vi "RPM probe test.vi"() -> ()   [LabVIEW 2016]
doc: "This example demonstrates how to write time-domain and frequency-domain data to a TDMS file using the Write to Measurement File Express VI."
uses:
  <vilib>/express/express analysis/Spectral/Block/exnSpectralBlock spectral measurements power poly.vi
  <vilib>/express/express analysis/Spectral/Block/exnSpectralBlock spectral measurements power DDT.vi
  <vilib>/express/express analysis/Spectral/XNode/ExpressSpectralMeasurementsBlockNode.xnode
panel:
  out "Boolean":bool
  in  "Dial":dbl(knob) scale=0.0..6500.0
  out "Measured Data":dynamicdata(graph)
  out "Power Spectrum":dynamicdata(graph)
  out "Scan number":i32
  in  "Stop":bool
  out "Value 2":i32 format="%_5f"
  # "Overview: Demonstrates how to write time-domain and frequency-domain data to a TDMS file using the Write to Measurement File Express VI.\nInstructions:\n1. Run the VI.\n2. Click Stop to stop the VI. The TDMS file will be displayed in the TDMS File Viewer.\n3. Delete the .tdms file (located at [LabVIEW Data]\\Example Time And Frequency Domain.tdms) when you are done."
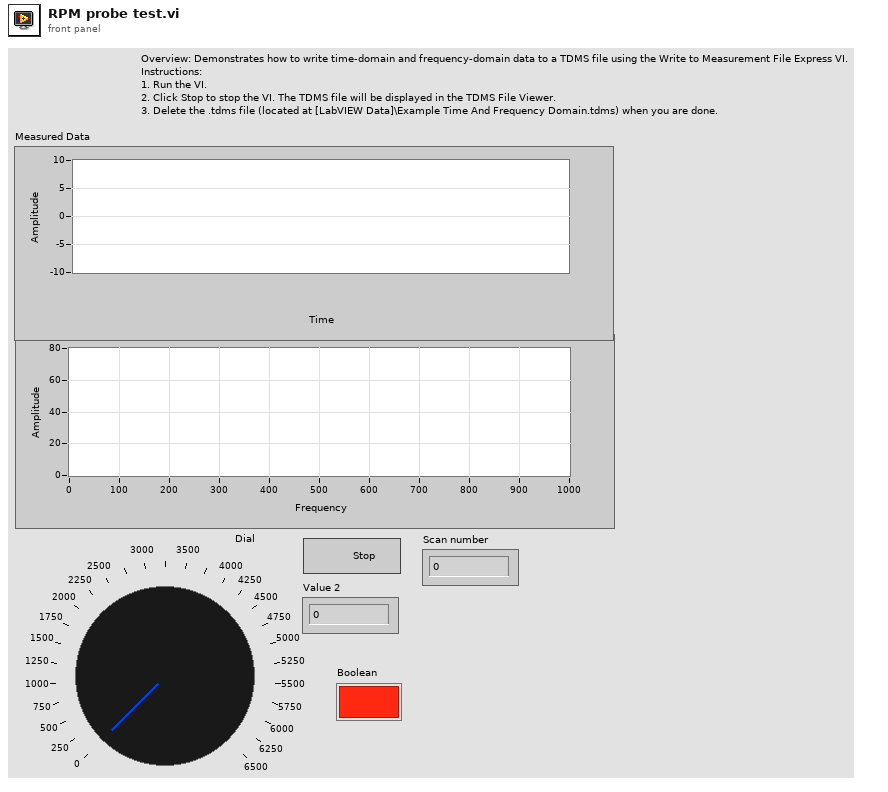
[diagram p1: front panel]
types:
  T1 = cluster{"averaging mode":u16, "weighting mode":u16, "number of averages":u32}
  T2 = cluster{"dB On (F)":bool, "unwrap phase (F)":bool, "convert to degree (F)":bool}
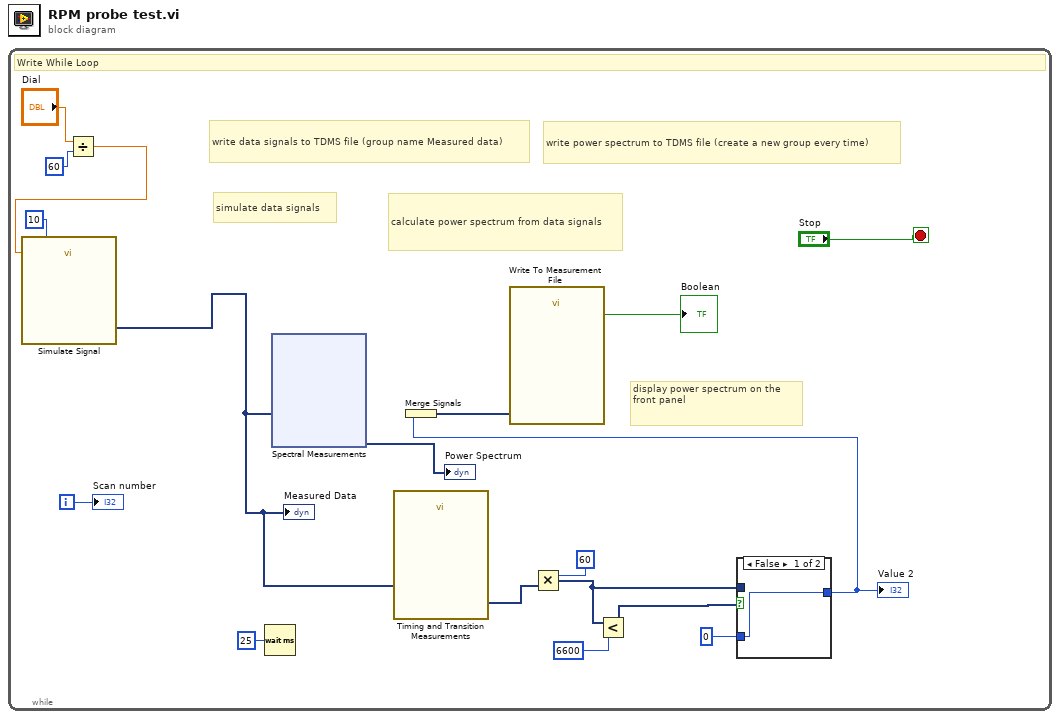
[diagram p0: block diagram]
diagram:
  n1 = while {
    i -> [w18]
    stop <- "Stop" stop-if-true
    # "simulate data signals"
    # "display power spectrum on the front panel"
    # "write power spectrum to TDMS file (create a new group every time)"
    # "calculate power spectrum from data signals"
    # "write data signals to TDMS file (group name Measured data)"
    # "Write While Loop"
    n2 = Divide(x="Dial", y=u32 60 ("milliseconds to wait")) -> (x/y=w6:dbl)
    n3 = call "Simulate Signal"("Frequency"=w6, "Amplitude"=u32 10 ("milliseconds to wait")) -> ("Square"=w11:dynamicdata)  [unwired: 5 in, 8 out]
    "Measured Data" <- w11
    n4 = Wait (ms)(milliseconds to wait=u32 25) -> ()  [unwired: 1 out]
    n5 = xnode "Spectral Measurements"("Signals"=w11) -> ("Power Spectrum"=→"Power Spectrum":dynamicdata)  [unwired: 1 in, 1 out]
    n6 = call "Timing and Transition Measurements"("Signals"=w11) -> ("Frequency"=w15:dynamicdata)  [unwired: 9 in, 1 out]
    n7 = Multiply(x=u32 60 ("milliseconds to wait"), y=w15) -> (x*y=w2:dynamicdata)
    n8 = Less?(x=w2, y=u32 6600 ("milliseconds to wait")) -> (x < y?=w4:dynamicdata)
    n9 = case shown="False" w4 {
      tunnel: u32 0 ("milliseconds to wait") -> [w19 _]
      tunnel: w2 -> [_ w20]
      tunnel: [w19 w20] -> w1
      frame False {
      }
      frame True {
      }
    }
    "Value 2" <- w1
    n10 = Merge Signals(w1) -> (w16:dynamicdata)
    n11 = call "Write To Measurement File"("Signals"=w16) -> ("Saving Data"=→"Boolean":bool)  [unwired: 16 in, 2 out]
    "Scan number" <- w18
  }
